vi "Send Acknowledge Message.vi"(0 "received message":T1, 5 "receiver port":u16, 9 "timeout":i32=10, 11 "error in":errorcluster) -> (10 "timed out?":bool, 15 "error out":errorcluster)   [LabVIEW 2013, in "AMC.lvlib"]
uses:
  AMC.lvlib
  Message.ctl
  <vilib>/NI/Tools/Keyed Array/KeyedArray.ctl
  Globals.vi
  <vilib>/NI/Tools/Keyed Array/Tools_KeyedArray.lvlib
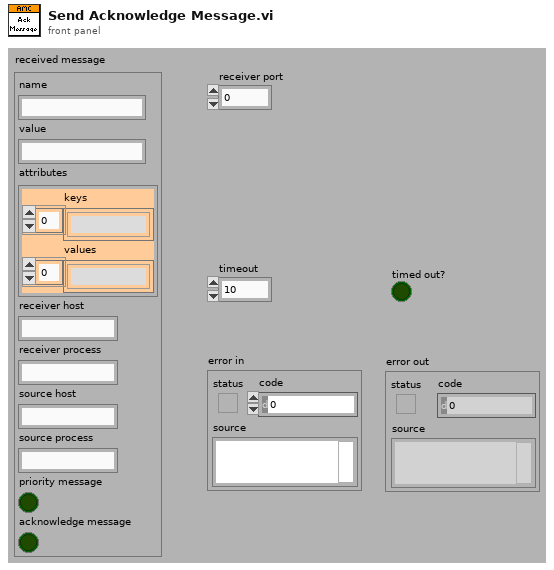
[diagram p1: front panel]
types:
  T1 = typedef "AMC.lvlib/Message.ctl" = cluster{"name":string, "value":string, "attributes":T2, "receiver host":string, "receiver process":string, "source host":string, "source process":string, "priority message":bool, "acknowledge message":bool}
  T2 = typedef "Tools_KeyedArray.lvlib/KeyedArray.ctl" = cluster{"keys":string[], "values":string[]}
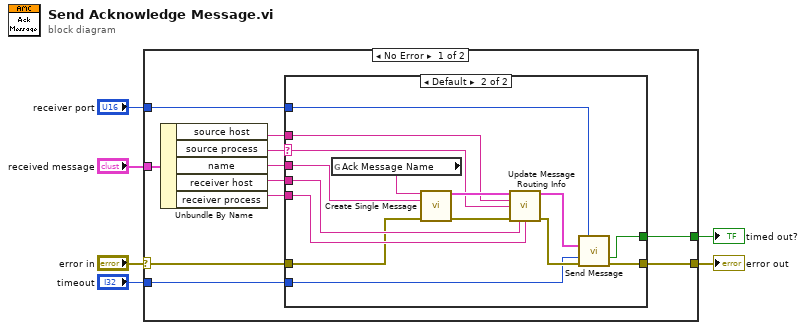
[diagram p0: block diagram]
diagram:
  n1 = case shown="No Error" "error in" {
    selector: "error in" -> [w10 w34]
    tunnel: "received message" -> [w17 _]
    tunnel: "receiver port" -> [w14 _]
    tunnel: [w15 w34] -> w3
    tunnel: "timeout" -> [w8 _]
    tunnel: [w7 _] -> w1
    frame No Error {
      n2 = Unbundle By Name(w17) -> ("source host"=w13:string, "source process"=w9:string, "name"=w16:string, "receiver host"=w12:string, "receiver process"=w11:string)
      n3 = case shown="Default" w9 {
        selector: w9 -> [_ w23]
        tunnel: w16 -> [_ w22]
        tunnel: [w18 w33] -> w15
        tunnel: w14 -> [_ w32]
        tunnel: w13 -> [_ w29]
        tunnel: w12 -> [_ w28]
        tunnel: w11 -> [_ w27]
        tunnel: w10 -> [w18 w25]
        tunnel: w8 -> [_ w21]
        tunnel: [_ w20] -> w7
        frame "" {
          # "There must be a source process name for an acknowledge message to be sent back to the source."
        }
        frame Default {
          n4 = global read "Globals.vi" "Ack Message Name"() -> (w19:string)
          n5 = call "Create Single Message.vi"("name"=w19, "value"=w22, "error in"=w25) -> ("message"=w31:T1, "error out"=w26:errorcluster)  [unwired: 11 in]
          n6 = call "Update Message Routing Info.vi"("message"=w31, "receiver host (\"\")"=w29, "receiver process (\"\")"=w23, "error in"=w26, "source host (\"\")"=w28, "source process (\"\")"=w27) -> ("message"=w30:T1, "error out"=w24:errorcluster)  [unwired: 8 in]
          n7 = call "Send Message.vi"("receiver port"=w32, "message"=w30, "timeout (-1 ms)"=w21, "error in"=w24) -> ("timed out?"=w20:bool, "error out"=w33:errorcluster)  [unwired: 9 in, 1 out]
        }
      }
    }
    frame Error {
    }
  }
  "error out" <- w3
  "timed out?" <- w1
